vi "get_LM_ID.vi"(8 "error in (no error)":errorcluster caption="错误输入（无错误）", 11 "LimitSwitch输入":refnum<class "LimitSwitch.lvclass">) -> (0 "error out":errorcluster caption="错误输出", 2 "LM ID":T1=1 items=["none", "S1", "S2", "S3"], 3 "LimitSwitch输出":refnum<class "LimitSwitch.lvclass">)   [LabVIEW 2016, in "MotionControl_UFO_3DOF.lvlib" / "LimitSwitch.lvclass"]
uses:
  <userlib>/MotionControl_UFO_3DOF/LimitSwitch/LimitSwitch.lvclass
  <userlib>/MotionControl_UFO_3DOF/LimitSwitch/LM_ID.ctl
  <userlib>/MotionControl_UFO_3DOF/LimitSwitch/LimitSwitch.lvclass/LimitSwitch.ctl
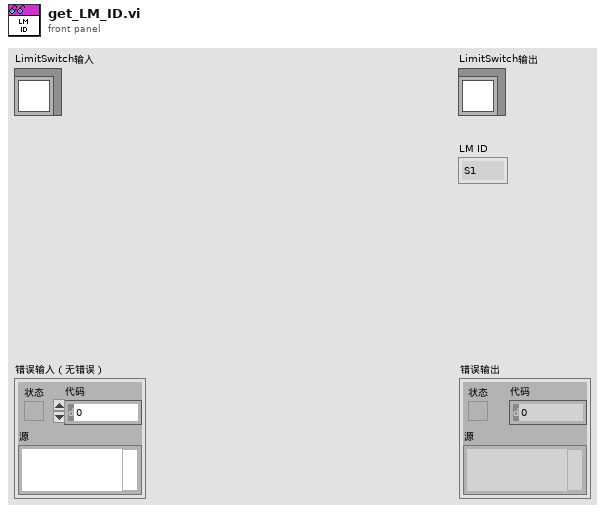
[diagram p1: front panel]
types:
  T1 = typedef "MotionControl_UFO_3DOF.lvlib/LimitSwitch.lvclass/LM_ID.ctl" = i32
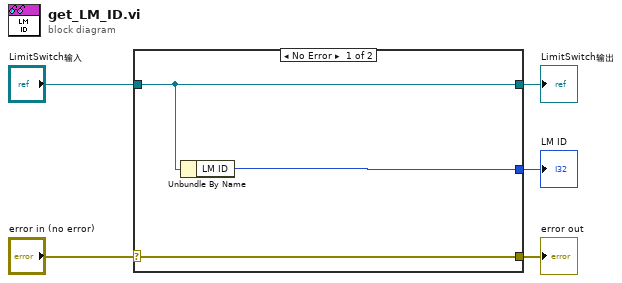
[diagram p0: block diagram]
diagram:
  n1 = case shown="No Error" "error in (no error)" {
    selector: "error in (no error)" -> [w8 w9]
    tunnel: [w8 w9] -> w4
    tunnel: [w7 w10] -> w2
    tunnel: "LimitSwitch输入" -> [w7 w10]
    tunnel: [w6 _] -> w1
    frame No Error {
      n2 = Unbundle By Name(w7) -> ("LM ID"=w6:T1)
    }
    frame Error {
    }
  }
  "error out" <- w4
  "LimitSwitch输出" <- w2
  "LM ID" <- w1
